vi "Dispatch Async Rx Transfer Groups.vi"(8 "error in (no error)":errorcluster, 9 "Plugin ID":i32, 10 "Dispatcher Interface in":refnum<class "Dispatcher Interface.lvclass">, 11 "Plugin in":refnum<class "Plugin.lvclass">) -> (0 "error out":errorcluster, 2 "Dispatcher Interface out":refnum<class "Dispatcher Interface.lvclass">, 3 "Plugin out":refnum<class "Plugin.lvclass">)   [LabVIEW 2017, in "DSF Core.lvlib" / "Plugin.lvclass"]
uses:
  Plugin.lvclass
  Timing/Timing.lvclass
  Transfer Group/Transfer Group.lvclass
  Interfaces/Dispatcher/Dispatcher Interface.lvclass
  Timing/Transfer Group Timing.lvclass
  C:/Git/DSF/Data Sharing Framework/Source/Core/Engine/Classes/Timing/Timing.lvclass
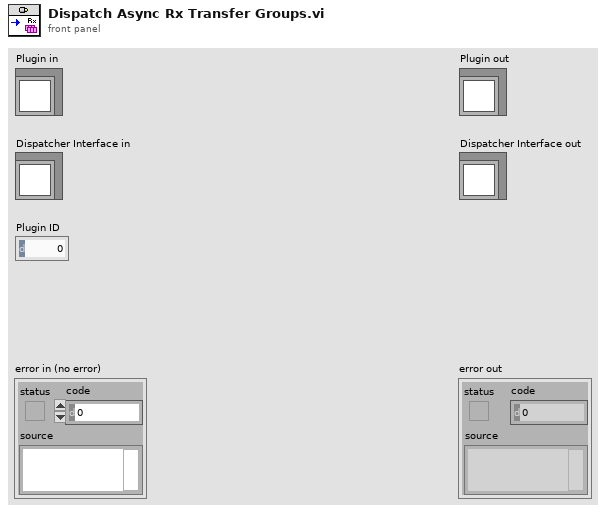
[diagram p1: front panel]
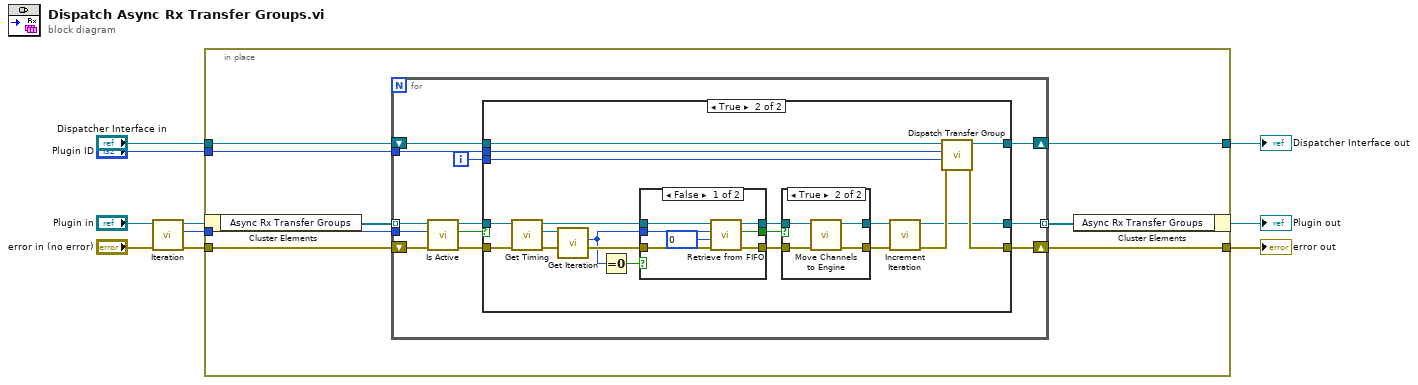
[diagram p0: block diagram]
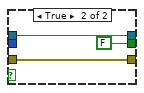
[diagram p3: hidden frame]
diagram:
  n1 = call "Iteration.vi"("Plugin in"="Plugin in") -> ("Iteration"=w6:u64, "Plugin out"=w7:refnum<class "Plugin.lvclass">)  [unwired: 9 in]
  n2 = in-place {
    in-place-border: w6 -> [w17]
    in-place-border: "error in (no error)" -> [w14]
    in-place-border: [w13] -> w8
    in-place-border: "Plugin ID" -> [w12]
    in-place-border: "Dispatcher Interface in" -> [w11]
    in-place-border: [w10] -> w2
    n3 = in-place-cluster #1(w7) -> ("Async Rx Transfer Groups"=w16:refnum<class "Transfer Group.lvclass">[])
    n4 = for {
      shift-right: [w28] -> w13
      shift-left: w14 -> [w27]
      tunnel: w16 -> [w26] mode=indexing
      tunnel: w17 -> [w25]
      tunnel: [w22] -> w15 mode=indexing
      shift-right: [w21] -> w10
      shift-left: w11 -> [w20]
      tunnel: w12 -> [w18]
      i -> [w19]
      n5 = call "Is Active.vi"("cycle count"=w25, "Transfer Group in"=w26) -> ("active this cycle?"=w24:bool, "Transfer Group out"=w23:refnum<class "Transfer Group.lvclass">)  [unwired: 8 in]
      n6 = case shown="True" w24 {
        tunnel: [w31 w37] -> w28
        tunnel: w27 -> [w31 w49]
        tunnel: w23 -> [w29 w41]
        tunnel: [w29 w32] -> w22
        tunnel: [w30 w35] -> w21
        tunnel: w20 -> [w30 w36]
        tunnel: w19 -> [_ w34]
        tunnel: w18 -> [_ w33]
        frame False {
        }
        frame True {
          n7 = call "Get Timing.vi"("Transfer Group in"=w41) -> ("Timing"=w48:refnum<class "Transfer Group Timing.lvclass">, "Transfer Group out"=w47:refnum<class "Transfer Group.lvclass">)  [unwired: 9 in]
          n8 = call "Get Iteration.vi"("Timing in"=w48) -> ("Iteration"=w40:u64)  [unwired: 9 in, 1 out]
          n9 = Equal To 0?(x=w40) -> (x = 0?=w39:bool)
          n10 = case shown="False" w39 {
            tunnel: w49 -> [w56 w59]
            tunnel: [w55 w57] -> w46
            tunnel: [w54 w59] -> w43
            tunnel: w47 -> [w53 w57]
            tunnel: w40 -> [w52 _]
            tunnel: [w51 FALSE ("iteration valid?")] -> w42
            frame False {
              n11 = call "Retrieve from FIFO.vi"("error in (no error)"=w56, "timeout in ms (0)"=0, "expected iteration"=w52, "Transfer Group in"=w53) -> ("error out"=w54:errorcluster, "iteration valid?"=w51:bool, "Transfer Group out"=w55:refnum<class "Transfer Group.lvclass">)  [unwired: 5 in]
            }
            frame True {
            }
          }
          n12 = case shown="True" w42 {
            tunnel: w46 -> [w61 w62]
            tunnel: [w61 w63] -> w45
            tunnel: [w60 w64] -> w44
            tunnel: w43 -> [w60 w65]
            frame False {
            }
            frame True {
              n13 = call "Move Channels to Engine.vi"("error in (no error)"=w65, "Transfer Group in"=w62) -> ("error out"=w64:errorcluster, "Transfer Group out"=w63:refnum<class "Transfer Group.lvclass">)  [unwired: 8 in]
            }
          }
          n14 = call "Increment Iteration.vi"("error in (no error)"=w44, "Transfer Group in"=w45) -> ("error out"=w38:errorcluster, "Transfer Group out"=w32:refnum<class "Transfer Group.lvclass">)  [unwired: 8 in]
          n15 = call "Dispatch Transfer Group.vi"("error in (no error)"=w38, "Transfer Group ID"=w34, "Plugin ID"=w33, "Dispatcher Interface in"=w36) -> ("error out"=w37:errorcluster, "Dispatcher Interface out"=w35:refnum<class "Dispatcher Interface.lvclass">)  [unwired: 6 in]
        }
      }
    }
    n16 = in-place-cluster #1("Async Rx Transfer Groups"=w15) -> (→"Plugin out":refnum<class "Plugin.lvclass">)
  }
  "error out" <- w8
  "Dispatcher Interface out" <- w2
